vi "test_Read I8 Register Value.vi"(8 "error in (no error)":errorcluster, 11 "TestCase in":refnum<class "FPGA Register IO Tests.lvclass">) -> (0 "error out":errorcluster, 3 "TestCase out":refnum<class "FPGA Register IO Tests.lvclass">)   [LabVIEW 2021, in "FPGA Register IO Tests.lvclass"]
uses:
  FPGA Register IO Tests.lvclass
  FPGA Register IO Tests.lvclass/FPGA Register IO Tests.ctl
  APIs/FPGA Register IO/Utilities/Find Register Offset.vi
  APIs/FPGA Register IO/SubVIs/Check Register Data Store.vi
  APIs/FPGA Register IO/Error Handling/Error 6001.vi
  APIs/FPGA Register IO/Error Handling/Error 6000.vi
  APIs/FPGA Register IO/Error Handling/Error 6002.vi
  APIs/FPGA Register IO/Error Handling/Error 6003.vi
  <vilib>/addons/_JKI Toolkits/VI Tester/TestCase.llb/TestCase.lvclass
  APIs/FPGA Register IO/FPGA Register IO.lvlib
  FPGA Addon Test Class/FPGA Addon Test Class.lvclass
  C:/Program Files/National Instruments/LabVIEW 2021/vi.lib/addons/_JKI Toolkits/VI Tester/TestCase.llb/TestCase.lvclass
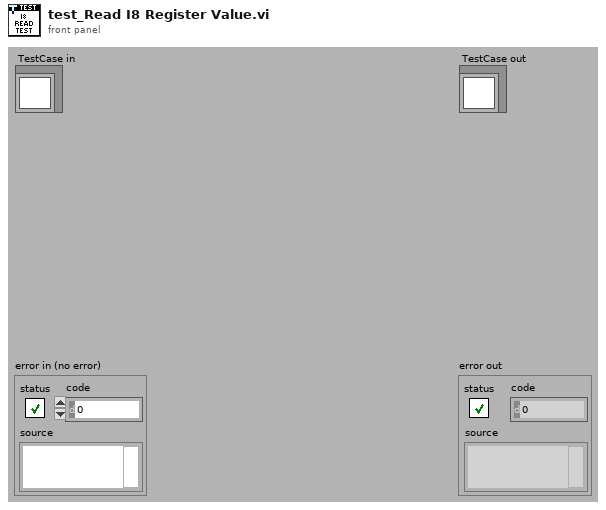
[diagram p1: front panel]
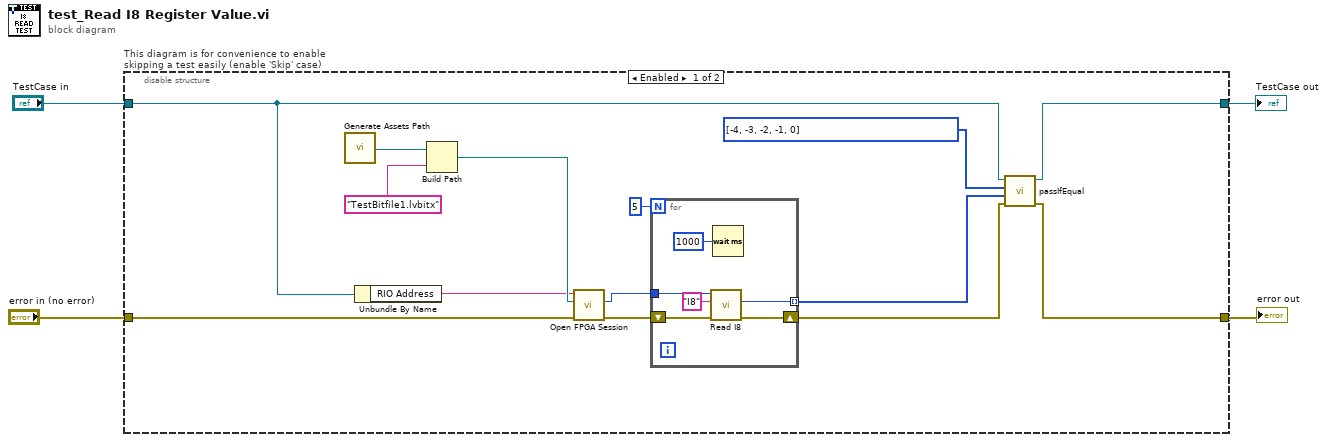
[diagram p0: block diagram]
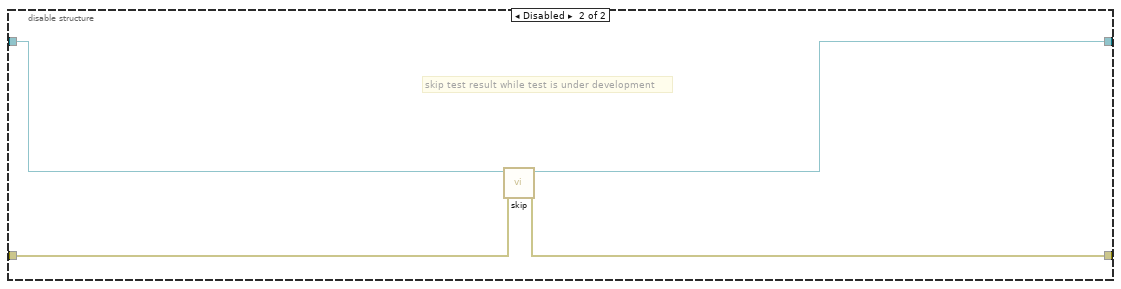
[diagram p2: hidden frame]
diagram:
  n1 = disable-structure "This diagram is for convenience to enable skipping a test easily (enable 'Skip' case)" shown="Enabled" {
    disable-tunnel: "TestCase in" -> [w9 w28]
    disable-tunnel: [w8 w26] -> w1
    disable-tunnel: [w7 w27] -> w3
    disable-tunnel: "error in (no error)" -> [w15 w25]
    frame Enabled {
      n2 = call "Generate Assets Path.vi"() -> ("Assets path"=w13:path)
      n3 = Unbundle By Name(w9) -> ("RIO Address"=w11:string)
      n4 = Build Path(base path=w13, name or relative path="TestBitfile1.lvbitx") -> (appended path=w12:path)
      n5 = call "Open FPGA Session.vi"("error in"=w15, "bitfile path"=w12, "device address"=w11) -> ("error out"=w18:errorcluster, "session out"=w17:u32)  [unwired: 6 in, 1 out]
      n6 = for {
        N: 5 -> [_]
        tunnel: w17 -> [w22]
        shift-right: [w23] -> w6
        shift-left: w18 -> [w24]
        tunnel: [w20] -> w5 mode=indexing
        n7 = call "Read I8.vi"("error in"=w24, "register name"="I8", "session in"=w22) -> ("error out"=w23:errorcluster, "value out"=w20:i8)  [unwired: 6 in, 1 out]
        n8 = Wait (ms)(milliseconds to wait=u32 1000) -> ()  [unwired: 1 out]
      }
      n9 = call-dynamic "passIfEqual.vi"("error in (no error)"=w6, "y"=w5, "x"=i8[] [-4, -3, -2, -1, 0] ("Array"), "TestCase in"=w9) -> ("error out"=w7:errorcluster, "TestCase out"=w8:refnum<class "FPGA Register IO Tests.lvclass">)  [unwired: 6 in]
    }
    frame Disabled {
      # "skip test result while test is under development"
      n10 = call <vilib>:"skip.vi"("error in (no error)"=w25, "TestCase in"=w28) -> ("error out"=w27:errorcluster, "TestCase out"=w26:refnum<class "FPGA Register IO Tests.lvclass">)  [unwired: 8 in]
    }
  }
  "error out" <- w3
  "TestCase out" <- w1
